vi "Priority.vi"(8 "error in (no error)":errorcluster, 11 "PathRegex Router in":refnum<class "PathRegex Router.lvclass">) -> (0 "error out":errorcluster, 2 "Priority":u16, 3 "PathRegex Router out":refnum<class "PathRegex Router.lvclass">)   [LabVIEW 2020, in "HTTP Server.lvlib" / "PathRegex Router.lvclass"]
uses:
  PathRegex Router.lvclass
  PathRegex Router.lvclass/PathRegex Router.ctl
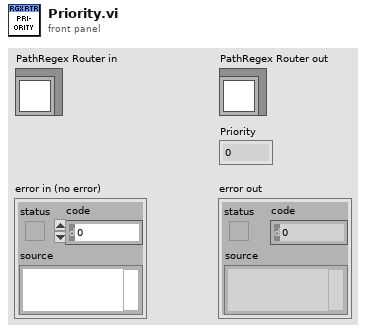
[diagram p1: front panel]
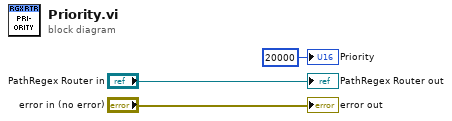
[diagram p0: block diagram]
diagram:
  "error out" <- "error in (no error)"
  "PathRegex Router out" <- "PathRegex Router in"
  "Priority" <- u16 20000 ("Priority")
